vi "Write equipoSeleccionado.vi"(8 "error in (no error)":errorcluster, 10 "equipoSeleccionado":string, 11 "Sonometro in":refnum<class "Sonometro.lvclass">) -> (0 "error out":errorcluster, 3 "Sonometro out":refnum<class "Sonometro.lvclass">)   [LabVIEW 2019, in "Sonometro.lvclass"]
uses:
  Sonometro.lvclass
  Equipo/Equipo.lvclass
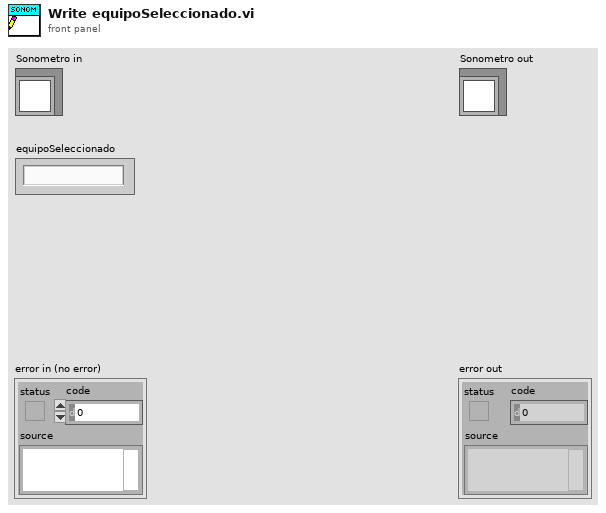
[diagram p1: front panel]
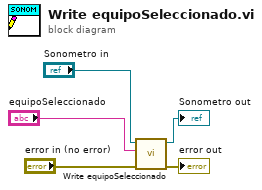
[diagram p0: block diagram]
diagram:
  n1 = call-parent "Write equipoSeleccionado.vi"("error in (no error)"="error in (no error)", "equipoSeleccionado"="equipoSeleccionado", "Equipo in"="Sonometro in") -> ("error out"=→"error out":errorcluster, "Equipo out"=→"Sonometro out":refnum<class "Sonometro.lvclass">)  [unwired: 7 in]
